vi "Impedance to Admittance.vi"(8 "Error In":errorcluster, 9 "Z (cplx)":T1 {"Z" format="%#_4g"}) -> (0 "Error Out":errorcluster, 1 "Y (complex)":T1 {"Z" format="%#_4g"})   [LabVIEW 2016]
uses:
  Trace (cplx).ctl
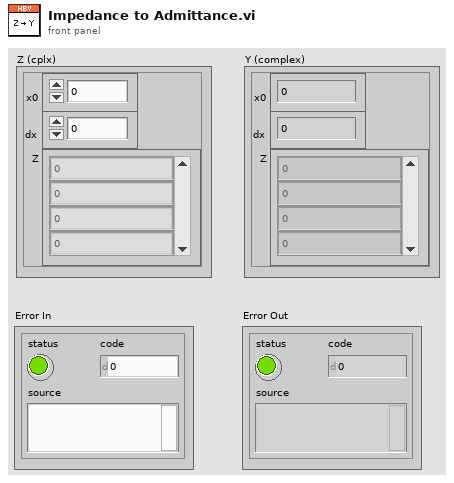
[diagram p1: front panel]
types:
  T1 = typedef "Trace (cplx).ctl" = cluster{"x0":dbl, "dx":dbl, "Z":cdb[]}
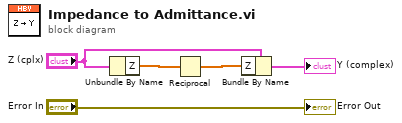
[diagram p0: block diagram]
diagram:
  n1 = Unbundle By Name("Z (cplx)") -> ("Z"=w3:cdb[])
  n2 = Reciprocal(x=w3) -> (1/x=w2:cdb[])
  n3 = Bundle By Name(cluster="Z (cplx)", "Z"=w2) -> (→"Y (complex)":T1)
  "Error Out" <- "Error In"
